vi "Fluence in Area.vi"(0 "Masked Image (I16only)":T2, 1 "Origin Image":i64[][](array[numeric]), 5 "Energie":dbl[unit], 7 "calibration mm/px":dbl[unit], 9 "Size of region":i32, 11 "error in (no error)":errorcluster) -> (6 "Fluence J/cm^2":dbl[unit], 8 "Energy in Area":dbl[unit], 10 "Max fluence area":T1, 14 "max value":i64, 15 "error out":errorcluster)   [LabVIEW 2014, in "Analyze.lvlib" / "Analyze Fluence.lvclass"]
uses:
  Analyze Fluence.lvclass
  <vilib>/vision/Image Controls.llb/IMAQ Image.ctl
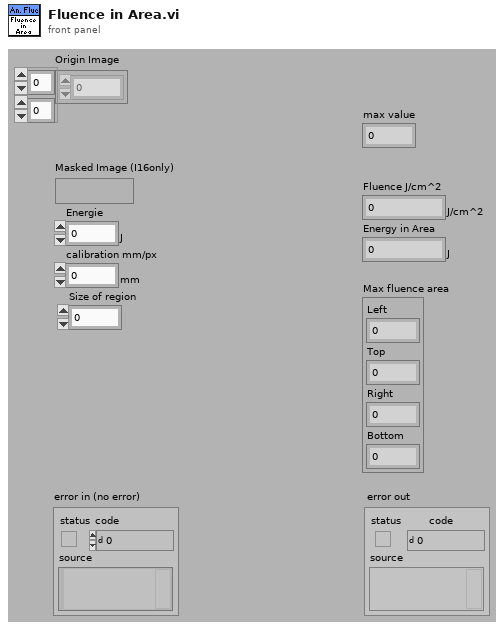
[diagram p1: front panel]
types:
  T1 = cluster{"Left":i32, "Top":i32, "Right":i32, "Bottom":i32}
  T2 = typedef "IMAQ Image.ctl" = refnum<image>
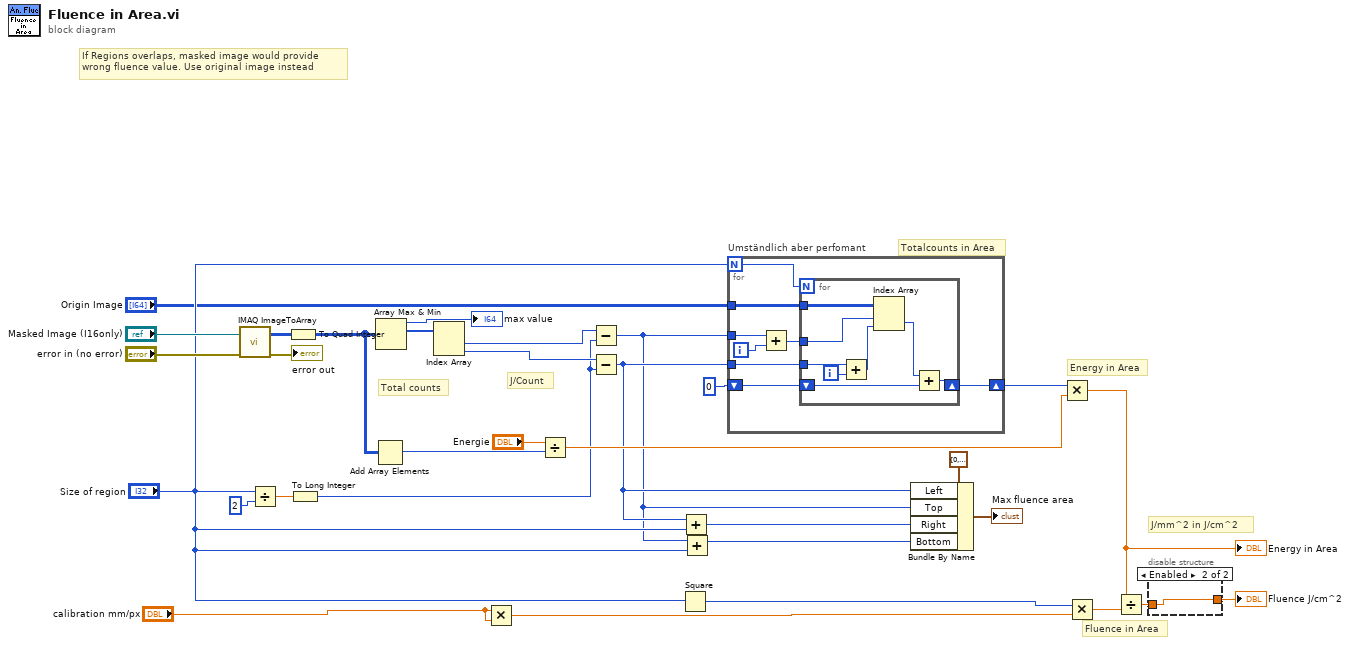
[diagram p0: block diagram]
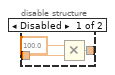
[diagram p2: hidden frame]
diagram:
  # "If Regions overlaps, masked image would provide \nwrong fluence value. Use original image instead"
  # "J/mm^2 in J/cm^2"
  # "Fluence in Area"
  # "Totalcounts in Area"
  # "Energy in Area"
  # "J/Count"
  # "Total counts"
  n1 = call "IMAQ ImageToArray"("error in (no error)"="error in (no error)", "Image"="Masked Image (I16only)") -> ("error out"=→"error out":errorcluster, "Image Pixels (I16)"=w10:i16[][])  [unwired: 2 in, 3 out]
  n2 = Divide(x="Size of region", y=u16 2) -> (x/y=w28:dbl)
  n3 = To Quad Integer(1:w10) -> (0:w9:i64[][])
  n4 = To Long Integer(number=w28) -> (32bit integer=w20:i32)
  n5 = Add Array Elements(numeric array=w9) -> (sum=w18:i64)
  n6 = Array Max & Min(array=w9) -> (max value=→"max value":i64, max index (indices)=w32:i32[])  [unwired: 2 out]
  n7 = Index Array(array=w32) -> (element #1=w29:i32, element #2=w27:i32)  [unwired: 2 in]
  n8 = Multiply(x="calibration mm/px", y="calibration mm/px") -> (x*y=w25:dbl[unit])
  n9 = Divide(x="Energie", y=w18) -> (x/y=w26:dbl[unit])
  n10 = Subtract(x=w29, y=w20) -> (x-y=w2:i32)
  n11 = Subtract(x=w27, y=w20) -> (x-y=w7:i32)
  n12 = Square(x="Size of region") -> (x^2=w24:i32)
  n13 = Add(x=w7, y="Size of region") -> (x+y=w16:i32)
  n14 = Add(x=w2, y="Size of region") -> (x+y=w17:i32)
  n15 = for "Umständlich aber perfomant" {
    N: "Size of region" -> [w33]
    tunnel: w2 -> [w39]
    tunnel: w7 -> [w40]
    shift-right: [w37] -> w4
    shift-left: i64 0 -> [w38]
    tunnel: "Origin Image" -> [w36]
    i -> [w34]
    n16 = Add(x=w39, y=w34) -> (x+y=w35:i32)
    n17 = for {
      N: w33 -> [_]
      tunnel: w40 -> [w44]
      tunnel: w35 -> [w48]
      shift-right: [w42] -> w37
      shift-left: w38 -> [w47]
      tunnel: w36 -> [w46]
      i -> [w45]
      n18 = Add(x=w44, y=w45) -> (x+y=w43:i32)
      n19 = Index Array(array=w46, index (row)=w48, index (col)=w43) -> (element=w41:i64)
      n20 = Add(x=w41, y=w47) -> (x+y=w42:i64)
    }
  }
  n21 = Bundle By Name(cluster=T1 {"Left"=0, "Top"=0, "Right"=0, "Bottom"=0} ("Rectangle"), "Left"=w7, "Top"=w2, "Right"=w16, "Bottom"=w17) -> (→"Max fluence area":T1)
  n22 = Multiply(x=w4, y=w26) -> (x*y=w19:dbl[unit])
  "Energy in Area" <- w19
  n23 = Multiply(x=w24, y=w25) -> (x*y=w23:dbl[unit])
  n24 = Divide(x=w19, y=w23) -> (x/y=w15:dbl[unit])
  n25 = disable-structure shown="Enabled" {
    disable-tunnel: w15 -> [w51 w52]
    disable-tunnel: [w50 w52] -> w14
    frame Disabled {
      n26 = Multiply(x=100.0, y=w51) -> (x*y=w50:dbl[unit])
    }
    frame Enabled {
    }
  }
  "Fluence J/cm^2" <- w14
